vi "ObtainGraphicsObject.vi"(8 "error in (no error)":errorcluster, 10 "Object Name":string, 11 "Scene in":refnum<vi>) -> (0 "error out":errorcluster, 2 "Found?":bool, 3 "Scene:New Object":refnum<vi>)   [LabVIEW 2014]
uses:
  <vilib>/picture/3D Picture Control/Object/Create Object (name).vi
  <vilib>/picture/3D Picture Control/NI_3D Picture Control.lvlib
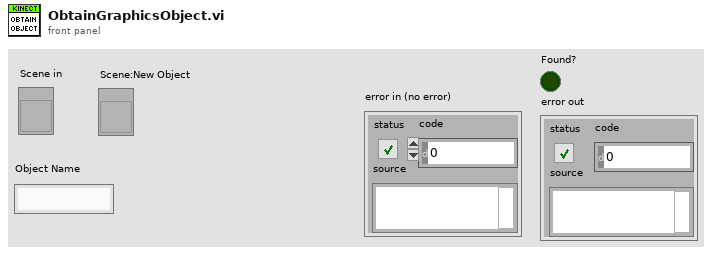
[diagram p1: front panel]
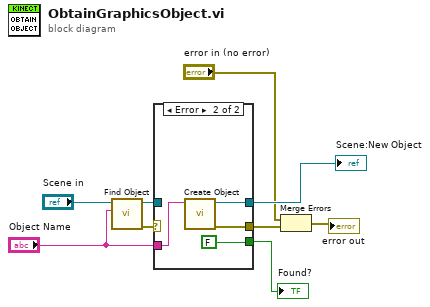
[diagram p0: block diagram]
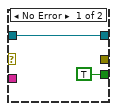
[diagram p2: hidden frame]
diagram:
  n1 = call <vilib>:"Find Object.vi"("Object Name"="Object Name", "Scene Refnum"="Scene in") -> ("error out"=w8:errorcluster, "Object Refnum"=w7:refnum<vi>)  [unwired: 8 in]
  n2 = case shown="Error" w8 {
    tunnel: [w11 w14] -> w5
    tunnel: w7 -> [w11 _]
    tunnel: "Object Name" -> [_ w15]
    tunnel: [TRUE FALSE] -> w4
    tunnel: [_ w12] -> w3
    frame No Error {
    }
    frame Error {
      n3 = call-poly <vilib>:"Create Object.vi"("Name"=w15) -> ("error out"=w12:errorcluster, "Scene:New Object"=w14:refnum<vi>)  [unwired: 9 in]
    }
  }
  "Scene:New Object" <- w5
  "Found?" <- w4
  n4 = Merge Errors("error in (no error)", w3) -> (→"error out":errorcluster)
